vi "Peakmap.vi"(8 "errin":errorcluster) -> (0 "error out":errorcluster, 3 "appended array":u32[](array[numeric]))   [LabVIEW 2020]
uses:
  <userlib>/PCAN Basic/Controls/Channel.ctl
  <userlib>/PCAN Basic/Controls/Parameter.ctl
  VarGLO/Global PEAK.vi
  <userlib>/PCAN Basic/PCANBasic.lvlib
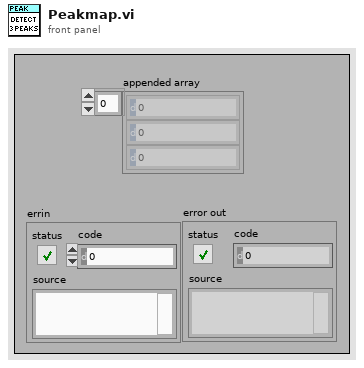
[diagram p1: front panel]
types:
  T1 = typedef "PCANBasic.lvlib/Channel.ctl" = enum16{"PCAN_NONEBUS", "not used1", "not used2", "not used3", "not used4", "not used5", "not used6", "not used7", "not used8", "not used9", "not used10", "not used11", "not used12", "not used13", "not used14", "not used15", "not used16", "not used17", "not used18", "not used19", "not used20", "not used21", "not used22", "not used23", "not used24", "not used25", "not used26", "not used27", "not used28", "not used29", "not used30", "not used31", "not used32", "PCAN_ISABUS1", "PCAN_ISABUS2", "PCAN_ISABUS3", "PCAN_ISABUS4", "PCAN_ISABUS5", "PCAN_ISABUS6", "PCAN_ISABUS7", "PCAN_ISABUS8", "not used41", "not used42", "not used43", "not used44", "not used45", "not used46", "not used47", "not used48", "PCAN_DNGBUS1", "not used50", "not used51", "not used52", "not used53", "not used54", "not used55", "not used56", "not used57", "not used58", "not used59", "not used60", "not used61", "not used62", "not used63", "not used64", "PCAN_PCIBUS1", "PCAN_PCIBUS2", "PCAN_PCIBUS3", "PCAN_PCIBUS4", "PCAN_PCIBUS5", "PCAN_PCIBUS6", "PCAN_PCIBUS7", "PCAN_PCIBUS8", "not used73", "not used74", "not used75", "not used76", "not used77", "not used78", "not used79", "not used80", "PCAN_USBBUS1", "PCAN_USBBUS2", "PCAN_USBBUS3", "PCAN_USBBUS4", "PCAN_USBBUS5", "PCAN_USBBUS6", "PCAN_USBBUS7", "PCAN_USBBUS8", "Not used89", "Not used90", "Not used91", "Not used92", "Not used93", "Not used94", "Not used95", "Not used96", "PCAN_PCCBUS1", "PCAN_PCCBUS2"}
  T2 = typedef "PCANBasic.lvlib/Parameter.ctl" = enum16{"Not Available", "PCAN device number", "PCAN 5-volt power", "PCAN receive event", "PCAN message filter", "PCAN API version", "PCAN channel version", "PCAN bus-off auto reset", "PCAN listen-only", "PCAN log location", "PCAN log status", "PCAN log configure", "PCAN log text", "PCAN channel condition", "PCAN hardware name"}
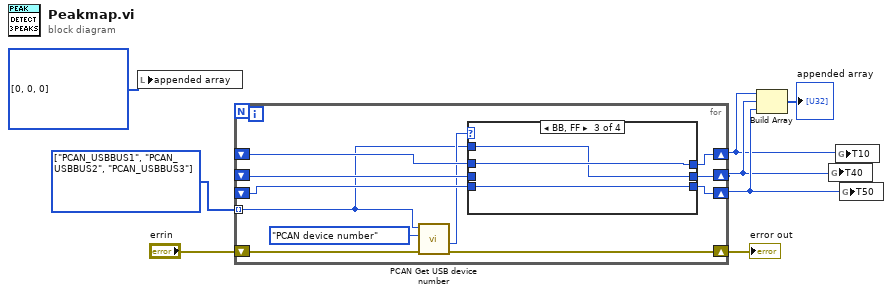
[diagram p0: block diagram]
diagram:
  w8 = T1[] [enum."PCAN_USBBUS1", enum."PCAN_USBBUS2", enum."PCAN_USBBUS3"] items=["PCAN_NONEBUS", "not used1", "not used2", "not used3", "not used4", "not used5", "not used6", "not used7", "not used8", "not used9", "not used10", "not used11", "not used12", "not used13", "not used14", "not used15", "not used16", "not used17", "not used18", "not used19", "not used20", "not used21", "not used22", "not used23", "not used24", "not used25", "not used26", "not used27", "not used28", "not used29", "not used30", "not used31", "not used32", "PCAN_ISABUS1", "PCAN_ISABUS2", "PCAN_ISABUS3", "PCAN_ISABUS4", "PCAN_ISABUS5", "PCAN_ISABUS6", "PCAN_ISABUS7", "PCAN_ISABUS8", "not used41", "not used42", "not used43", "not used44", "not used45", "not used46", "not used47", "not used48", "PCAN_DNGBUS1", "not used50", "not used51", "not used52", "not used53", "not used54", "not used55", "not used56", "not used57", "not used58", "not used59", "not used60", "not used61", "not used62", "not used63", "not used64", "PCAN_PCIBUS1", "PCAN_PCIBUS2", "PCAN_PCIBUS3", "PCAN_PCIBUS4", "PCAN_PCIBUS5", "PCAN_PCIBUS6", "PCAN_PCIBUS7", "PCAN_PCIBUS8", "not used73", "not used74", "not used75", "not used76", "not used77", "not used78", "not used79", "not used80", "PCAN_USBBUS1", "PCAN_USBBUS2", "PCAN_USBBUS3", "PCAN_USBBUS4", "PCAN_USBBUS5", "PCAN_USBBUS6", "PCAN_USBBUS7", "PCAN_USBBUS8", "Not used89", "Not used90", "Not used91", "Not used92", "Not used93", "Not used94", "Not used95", "Not used96", "PCAN_PCCBUS1", "PCAN_PCCBUS2"]
  n1 = local write "appended array"(u32[] [0, 0, 0] ("appended array")) -> ()
  n2 = for {
    tunnel: w8 -> [w9] mode=indexing
    shift-right: [w18] -> w3
    shift-left: _ -> [w13]
    shift-right: [w17] -> w4
    shift-left: _ -> [w14]
    shift-right: [w16] -> w5
    shift-left: _ -> [w15]
    shift-right: [w11] -> w7
    shift-left: "errin" -> [w12]
    n3 = call <userlib>:"PCAN Get USB device number.vi"("error in (no error)"=w12, "Parameter"=Parameter."PCAN device number", "Channel"=w9) -> ("error out"=w11:errorcluster, "PCAN Device Number"=w10:u32)  [unwired: 6 in, 1 out]
    n4 = case shown="BB, FF" w10 {
      tunnel: [w22 w23 w27 w31] -> w18
      tunnel: [w21 w25 w26 w30] -> w17
      tunnel: [w20 w24 w28 w29] -> w16
      tunnel: w14 -> [w21 w25 _ w30]
      tunnel: w15 -> [w20 w24 w28 _]
      tunnel: w13 -> [w22 _ w27 w31]
      tunnel: w9 -> [_ w23 w26 w29]
      frame 0, Default {
      }
      frame 170 {
      }
      frame 187, 255 {
      }
      frame 204 {
      }
    }
  }
  "error out" <- w7
  n5 = Build Array(w3, w4, w5) -> (→"appended array":T1[])
  n6 = global write "Global PEAK.vi" "T40"(w4) -> ()
  n7 = global write "Global PEAK.vi" "T10"(w3) -> ()
  n8 = global write "Global PEAK.vi" "T50"(w5) -> ()
